vi "Checksum for Command.vi"(10 "Message":string, 11 "Address":i32) -> (3 "Formated Message":string)   [LabVIEW 2018, in "Huber Unistat 410 TCU.lvlib"]
uses:
  Huber Unistat 410 TCU.lvlib
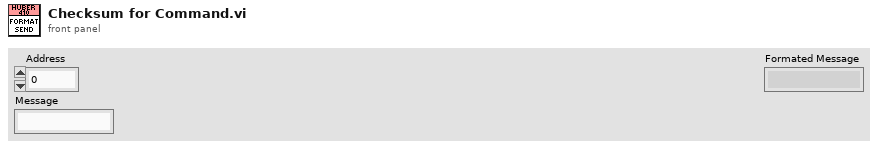
[diagram p1: front panel]
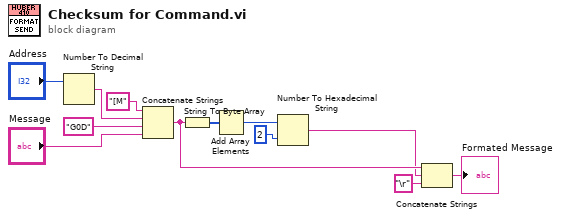
[diagram p0: block diagram]
diagram:
  n1 = Number To Decimal String(number="Address") -> (decimal integer string=w8:string)  [unwired: 1 in]
  n2 = Concatenate Strings("[M" ("string"), w8, "G0D" ("string"), "Message") -> (w4:string)
  n3 = String To Byte Array(string=w4) -> (unsigned byte array=w12:u8[])
  n4 = Add Array Elements(numeric array=w12) -> (sum=w11:u8)
  n5 = Number To Hexadecimal String(1:i16 2 ("width (-)"), 2:w11) -> (0:w3:string)
  n6 = Concatenate Strings(w4, w3, "\r" ("string")) -> (→"Formated Message":string)
